vi "Daten fuer LogFile sepparieren.vi"(8 "Messwerte":sgl[](array[numeric]), 10 "labBaseName":string, 11 "Aktuelle Gasliste gesamt":T1[](array[typedef])) -> (0 "Array für LogFile":sgl[](array[numeric]), 3 "Gasliste für LogFile":T1[](array[typedef]))   [LabVIEW 2020, in "Messdaten.lvlib"]
uses:
  Messdaten.lvlib
  Visualisierungs Elemente/String - Ausgabefeld.ctl
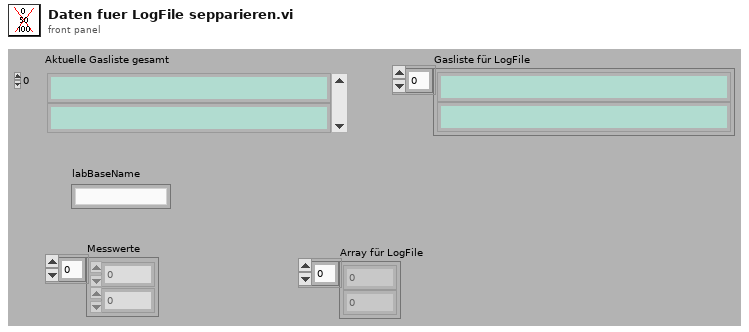
[diagram p1: front panel]
types:
  T1 = typedef "String - Ausgabefeld.ctl" = string
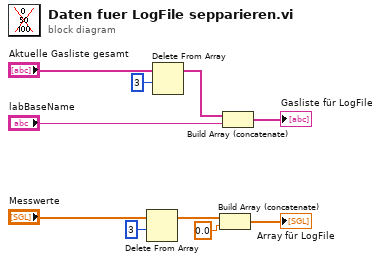
[diagram p0: block diagram]
diagram:
  n1 = Delete From Array(array="Messwerte", length=3 ("Länge")) -> (array with subset deleted=w5:sgl[])  [unwired: 1 in, 1 out]
  n2 = Delete From Array(array="Aktuelle Gasliste gesamt", length=3 ("Länge")) -> (array with subset deleted=w2:T1[])  [unwired: 1 in, 1 out]
  n3 = Build Array (concatenate)(w5, sgl 0.0) -> (→"Array für LogFile":sgl[])
  n4 = Build Array (concatenate)(w2, "labBaseName") -> (→"Gasliste für LogFile":T1[])
